vi "Action Stop Pump.vi"(5 "Retry Attempts (0)":i32 min=0, 7 "Fast Comms (F)":bool, 8 "error in":errorcluster, 11 "VISA resource name":refnum<visa-resource-name>) -> (0 "error out":errorcluster, 3 "VISA resource name out":refnum<visa-resource-name>)   [LabVIEW 2020, in "ChromTech MX-Class Drivers.lvlib"]
doc: "Stop the pump."
uses:
  <instrlib>/RxnRover/ChromtechNextGenDriver/ChromTech MX-Class Drivers.lvlib
panel:
  out "Response":string
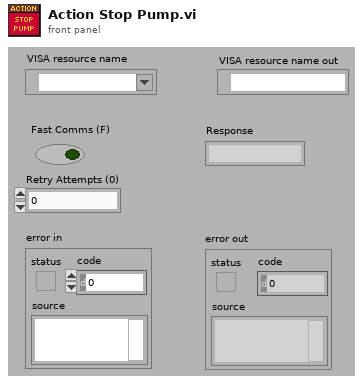
[diagram p1: front panel]
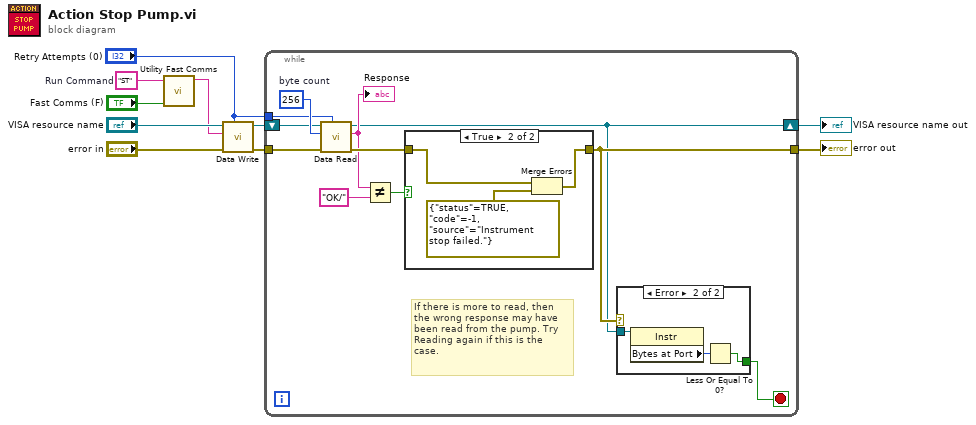
[diagram p0: block diagram]
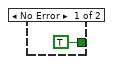
[diagram p2: hidden frame]
diagram:
  w7 = "ST"  # Run Command
  n1 = call <instrlib>:"Utility Fast Comms.vi"("Fast Comms"="Fast Comms (F)", "Command"=w7) -> ("Fast Command"=w6:string)  [unwired: 9 in]
  n2 = call <instrlib>:"Data Write.vi"("Retry Attempts (0)"="Retry Attempts (0)", "error in (no error)"="error in", "Command"=w6, "VISA Refnum in"="VISA resource name") -> ("error out"=w5:errorcluster, "VISA Refnum out"=w4:refnum<visa-resource-name>)  [unwired: 6 in]
  n3 = while {
    tunnel: "Retry Attempts (0)" -> [w14]
    shift-right: [w12] -> w1
    shift-left: w4 -> [w16]
    tunnel: w5 -> [w17]
    tunnel: [w13] -> w2
    stop <- w11 stop-if-true
    w21 = u32 256  # byte count
    # "If there is more to read, then\nthe wrong response may have\nbeen read from the pump. Try\nReading again if this is the\ncase."
    n4 = call <instrlib>:"Data Read.vi"("Retry Attempts (0)"=w14, "error in (no error)"=w17, "Bytes to read"=w21, "VISA Refnum in"=w16) -> ("error out"=w18:errorcluster, "read buffer"=w15:string, "VISA Refnum out"=w12:refnum<visa-resource-name>)  [unwired: 5 in]
    "Response" <- w15
    n5 = Not Equal?(x=w15, y="OK/") -> (x != y?=w19:bool)
    n6 = case shown="True" w19 {
      tunnel: [w26 w28] -> w13
      tunnel: w18 -> [w26 w27]
      frame False {
      }
      frame True {
        n7 = Merge Errors(w27, errorcluster {"status"=TRUE, "code"=-1, "source"="Instrument stop failed."} ("error out")) -> (w28:errorcluster)
      }
    }
    n8 = case shown="Error" w13 {
      tunnel: w12 -> [_ w25]
      tunnel: [TRUE w23] -> w11
      frame No Error {
      }
      frame Error {
        n9 = property class="Instr"(reference=w25) -> ("Bytes at Port"=w24:u32)  [unwired: 1 in, 2 out]
        n10 = Less Or Equal To 0?(x=w24) -> (x <= 0?=w23:bool)
      }
    }
  }
  "VISA resource name out" <- w1
  "error out" <- w2
